vi "ROTATION SELECT.vi"(10 "POVs in":i16[](array[numeric]), 11 "TWIST in":dbl=0.5) -> (3 "Jr":dbl=-0.32666666666666666)   [LabVIEW 2023]
uses:
  ctrl defs/ctrl pivot select.ctl
  Global odometry.vi
  <vilib>/express/express arith-compare/Formula/XNode/ExpressFormulaBlockNode.xnode
panel:
  out "select pivot point":T1
  in  "testing":bool
  in  "Spin\nMIN scale":dbl=0.15 format="%#_13g"
  out "twist pre-out":dbl=0.005
  out "twist out":dbl=-0.32666666666666666
  in  "Spin\nMAX":dbl=1.0 format="%#_13g"
  in  "Max dx/dt\nTWIST":dbl=5.0
  in  "deadband\nTWIST":dbl=0.25 format="%#_13g"
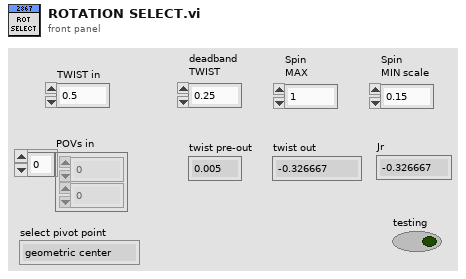
[diagram p1: front panel]
types:
  T1 = typedef "ctrl pivot select.ctl" = enum16{"geometric center", "CG", "FL", "FR", "RR", "RL", "other"}
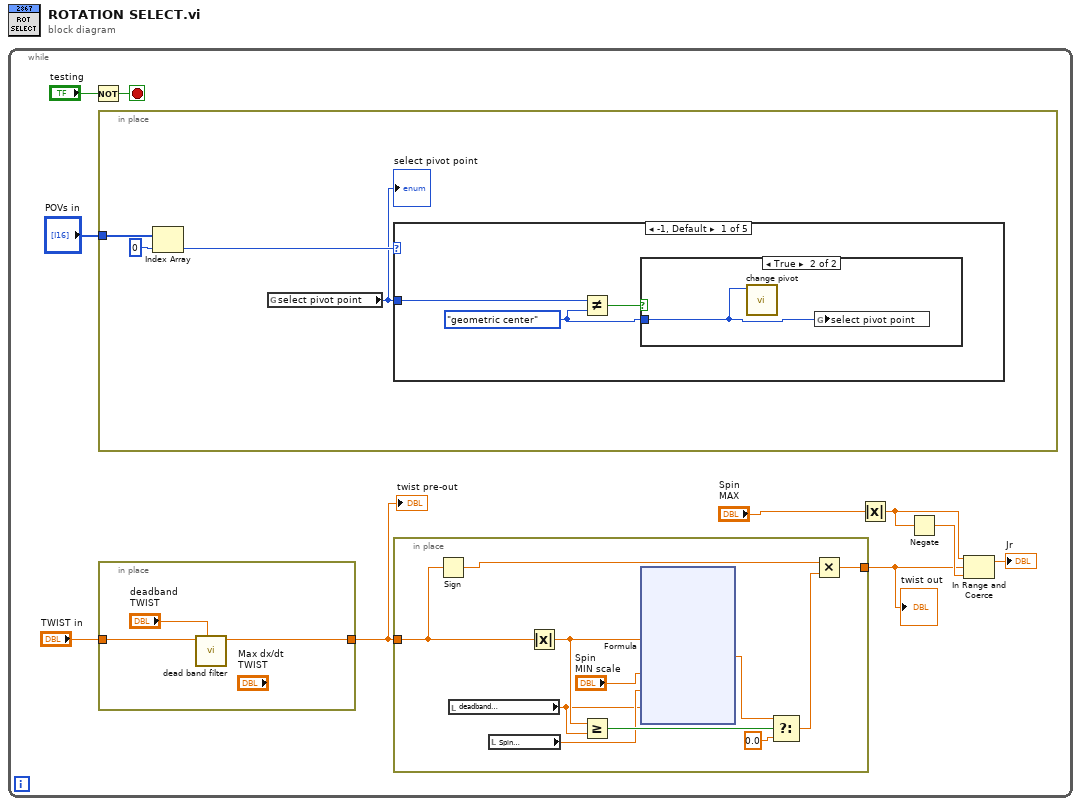
[diagram p0: block diagram]
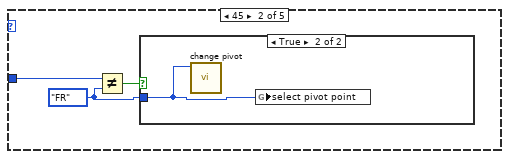
[diagram p3: hidden frame]
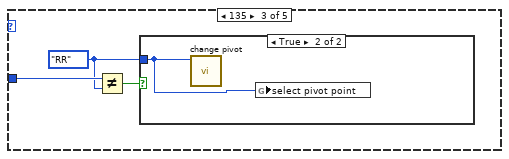
[diagram p5: hidden frame]
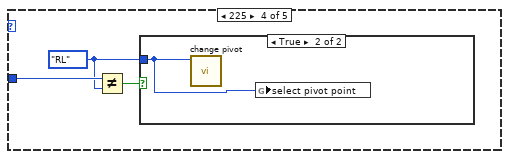
[diagram p7: hidden frame]
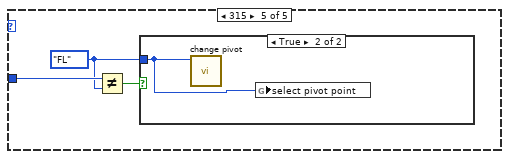
[diagram p9: hidden frame]
diagram:
  n1 = while {
    stop <- w3 stop-if-true
    n2 = Not(x="testing") -> (.not. x?=w3:bool)
    n3 = in-place {
      in-place-border: "POVs in" -> [w37]
      n4 = Index Array(array=w37, index=0) -> (element=w38:i16)
      n5 = global read "Global odometry.vi" "select pivot point"() -> (w36:T1)
      "select pivot point" <- w36
      n6 = case shown="-1, Default" w38 {
        tunnel: w36 -> [w41 w45 w49 w53 w57]
        frame -1, Default {
          w40 = ctrl_pivot_select."geometric center" ("select pivot point")
          n7 = Not Equal?(x=w41, y=w40) -> (x != y?=w42:bool)
          n8 = case shown="True" w42 {
            tunnel: w40 -> [_ w43]
            frame False {
            }
            frame True {
              n9 = call "change pivot.vi"("select pivot point"=w43) -> ()  [unwired: 10 in, 1 out]
              n10 = global write "Global odometry.vi" "select pivot point"(w43) -> ()
            }
          }
        }
        frame 45 {
          w44 = ctrl_pivot_select."FR" ("select pivot point")
          n11 = Not Equal?(x=w45, y=w44) -> (x != y?=w46:bool)
          n12 = case shown="True" w46 {
            tunnel: w44 -> [_ w47]
            frame False {
            }
            frame True {
              n13 = call "change pivot.vi"("select pivot point"=w47) -> ()  [unwired: 10 in, 1 out]
              n14 = global write "Global odometry.vi" "select pivot point"(w47) -> ()
            }
          }
        }
        frame 135 {
          w48 = ctrl_pivot_select."RR" ("select pivot point")
          n15 = Not Equal?(x=w49, y=w48) -> (x != y?=w50:bool)
          n16 = case shown="True" w50 {
            tunnel: w48 -> [_ w51]
            frame False {
            }
            frame True {
              n17 = call "change pivot.vi"("select pivot point"=w51) -> ()  [unwired: 10 in, 1 out]
              n18 = global write "Global odometry.vi" "select pivot point"(w51) -> ()
            }
          }
        }
        frame 225 {
          w52 = ctrl_pivot_select."RL" ("select pivot point")
          n19 = Not Equal?(x=w53, y=w52) -> (x != y?=w54:bool)
          n20 = case shown="True" w54 {
            tunnel: w52 -> [_ w55]
            frame False {
            }
            frame True {
              n21 = call "change pivot.vi"("select pivot point"=w55) -> ()  [unwired: 10 in, 1 out]
              n22 = global write "Global odometry.vi" "select pivot point"(w55) -> ()
            }
          }
        }
        frame 315 {
          w56 = ctrl_pivot_select."FL" ("select pivot point")
          n23 = Not Equal?(x=w57, y=w56) -> (x != y?=w58:bool)
          n24 = case shown="True" w58 {
            tunnel: w56 -> [_ w59]
            frame False {
            }
            frame True {
              n25 = call "change pivot.vi"("select pivot point"=w59) -> ()  [unwired: 10 in, 1 out]
              n26 = global write "Global odometry.vi" "select pivot point"(w59) -> ()
            }
          }
        }
      }
    }
    n27 = in-place {
      in-place-border: [w61] -> w6
      in-place-border: "TWIST in" -> [w60]
      n28 = call "dead band filter.vi"("deadband"="deadband\nTWIST", "input"=w60) -> ("output"=w61:dbl)  [unwired: 9 in]
    }
    "twist pre-out" <- w6
    n29 = in-place {
      in-place-border: w6 -> [w21]
      in-place-border: [w16] -> w5
      n30 = Sign(1:w21) -> (0:w17:dbl)
      n31 = local read "deadband\nTWIST"() -> (w12:dbl)
      n32 = local read "Spin\nMAX"() -> (w13:dbl)
      n33 = Absolute Value(x=w21) -> (abs(x)=w15:dbl)
      n34 = Greater Or Equal?(x=w15, y=w12) -> (x >= y?=w20:bool)
      n35 = xnode "Formula"("x"=w15, "min"="Spin\nMIN scale", "max"=w13, "dB"=w12) -> ("Result"=w11:dbl)  [unwired: 1 in, 1 out]
      n36 = Select(t=w11, s=w20, f=0.0) -> (s? t:f=w18:dbl)
      n37 = Multiply(x=w17, y=w18) -> (x*y=w16:dbl)
    }
    "twist out" <- w5
    n38 = Absolute Value(x="Spin\nMAX") -> (abs(x)=w2:dbl)
    n39 = Negate(x=w2) -> (-x=w7:dbl)
    n40 = In Range and Coerce(upper limit=w2, x=w5, lower limit=w7) -> (coerced(x)=→"Jr":dbl)  [unwired: 1 out]
  }
